vi "Stop Core.vi"(10 "final error code":i32, 11 "Actor_NI6008 in":refnum<class "Actor_NI6008.lvclass">) -> (3 "Actor_NI6008 out":refnum<class "Actor_NI6008.lvclass">)   [LabVIEW 2020, in "Actor_NI6008.lvlib" / "Actor_NI6008.lvclass"]
doc: "(<B>Filename</B>: Actor Framework.lvlib:Actor.lvclass:Stop Core.vi)\n\nDefines what the actor does before it stops. Use the <B>final error code</B> input to determine whether the actor shut down in response to an error.\n\nBy default, this method passes the Stop message along to all auto-stop nested actors. A descendant class may override this method to define additional behavior, such as shutting down any processes the actor initiated in its override of the Actor Core method."
uses:
  Actor_NI6008.lvclass
  Actor_NI6008.lvclass/Actor_NI6008.ctl
  <vilib>/ActorFramework/Actor/Actor.lvclass
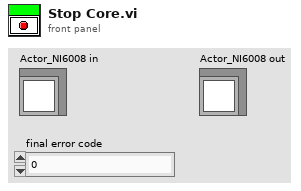
[diagram p1: front panel]
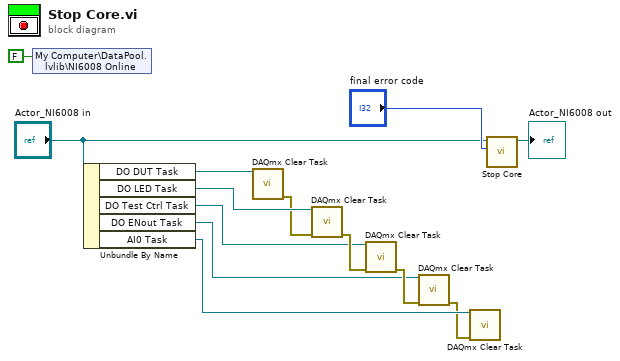
[diagram p0: block diagram]
diagram:
  n1 = shared-variable "My Computer\\DataPool.lvlib\\NI6008 Online"(FALSE ("NI6008 Online")) -> ()  [unwired: 1 in, 1 out]
  n2 = Unbundle By Name("Actor_NI6008 in") -> ("DO DUT Task"=w10:refnum<k21>, "DO LED Task"=w8:refnum<k21>, "DO Test Ctrl Task"=w5:refnum<k21>, "DO ENout Task"=w3:refnum<k21>, "AI0 Task"=w2:refnum<k21>)
  n3 = call <vilib>:"DAQmx Clear Task.vi"("task in"=w10) -> ("error out"=w7:errorcluster)  [unwired: 14 in]
  n4 = call <vilib>:"DAQmx Clear Task.vi"("task in"=w8, "error in"=w7) -> ("error out"=w6:errorcluster)  [unwired: 13 in]
  n5 = call <vilib>:"DAQmx Clear Task.vi"("task in"=w5, "error in"=w6) -> ("error out"=w4:errorcluster)  [unwired: 13 in]
  n6 = call <vilib>:"DAQmx Clear Task.vi"("task in"=w3, "error in"=w4) -> ("error out"=w1:errorcluster)  [unwired: 13 in]
  n7 = call <vilib>:"DAQmx Clear Task.vi"("task in"=w2, "error in"=w1) -> ()  [unwired: 13 in, 1 out]
  n8 = call-parent "Stop Core.vi"("final error code"="final error code", "Actor in"="Actor_NI6008 in") -> ("Actor out"=→"Actor_NI6008 out":refnum<class "Actor_NI6008.lvclass">)  [unwired: 9 in]
